vi "CPP_CalcTubingCorrection.vi"() -> (5 "Plug in titles":string[](array[string]), 7 "Plug in values":string[](array[string]))   [LabVIEW 2010]
uses:
  Globals/Plug_in_data_global.vi
  Globals/Meas_global.vi
  <vilib>/Analysis/NI_AALPro.lvlib
  <vilib>/Analysis/NI_AALBase.lvlib
panel:
  out "df":dbl format="%0.2f"
  out "Spectra":cluster{dbl, "df":dbl, dbl[][]}(graph)
  out "Current Block No":i32
  in  "stop":bool
  out "Time Traces":cluster{dbl, dbl, dbl[][]}(graph)
  in  "TestXducer":u16(ring) items=["Gen (Ref)", "Gen (t5w1)", "Gen (t2w2)", "Gen (t1w5)"]
  in  "RefXducer":u16(ring) items=["Gen (Ref)", "Gen (t5w1)", "Gen (t2w2)", "Gen (t1w5)"]
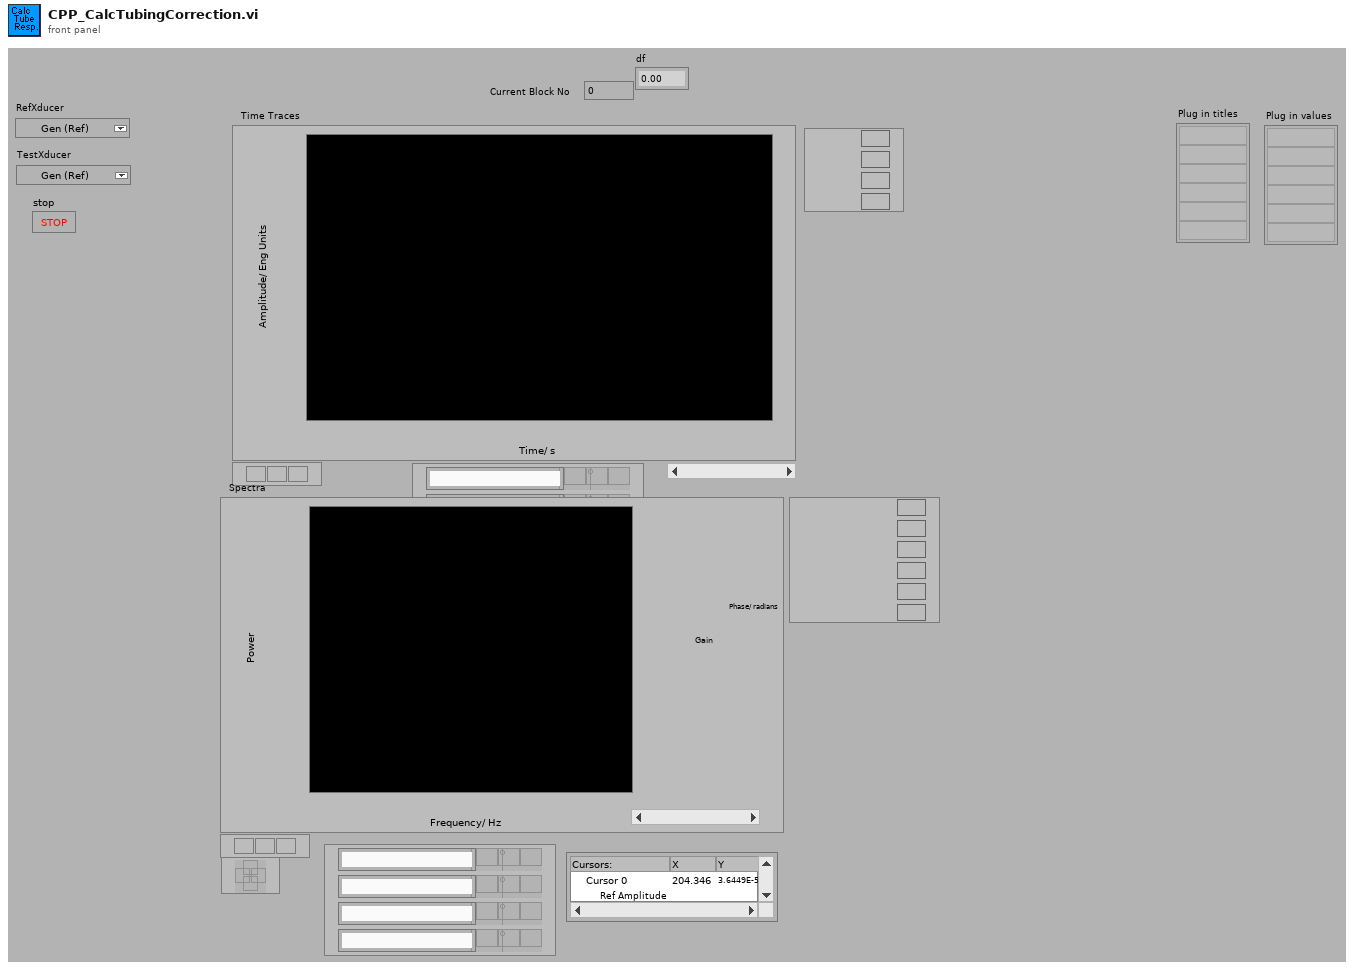
[diagram p1: front panel]
types:
  T1 = typedef "Analysis_info_cluster.ctl" = cluster{"Colour":u32, "Inst type":T2, "Inst name":string, "Symbol":string, "Code name":string, "Extra Info":string, "Inst Array":T3, "Index":i32, "Voltage Index":i32, "Extra Titles":string[], "Extra Values":string[]}
  T2 = typedef "Inst_type.ctl" = enum16{"Propeller anemometer", "Raw voltage", "Pressure Transducer", "Pitot-static tube", "Preston tube", "Hot wire", "Cross wire 1", "Cross wire 2", "Generic Linear", "Generic Polynomial", "Generic BackPoly", "Fast FID", "Thermocouple", "Cold wire", "Pulsed Wire", "LDA Vel", "LDA Tran time", "LDA Arr time"}
  T3 = typedef "Instrument_Array.ctl" = enum16{"PWA", "LDA", "Analogue"}
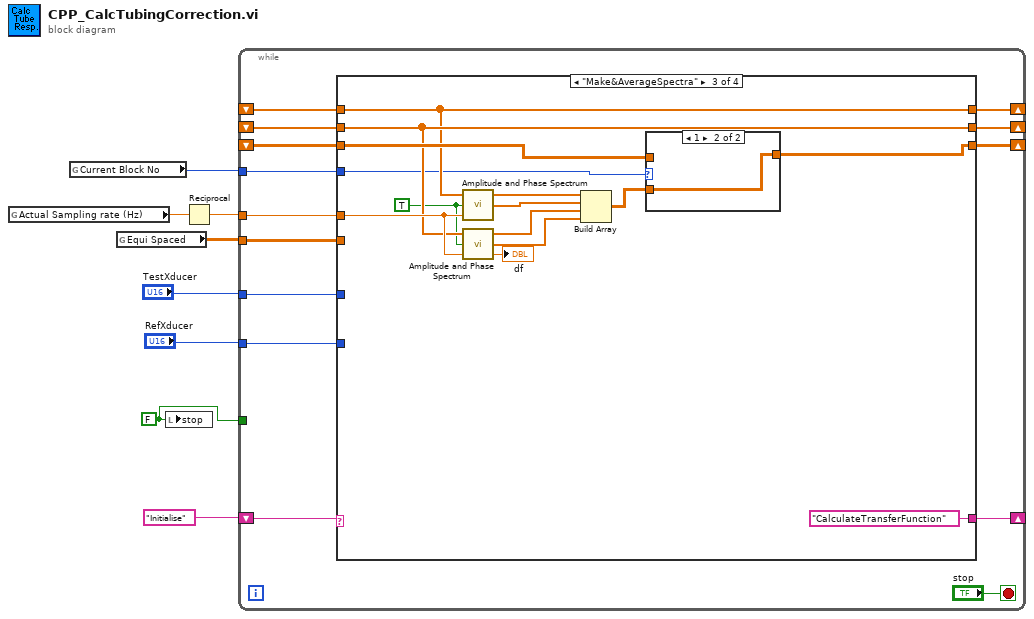
[diagram p0: block diagram]
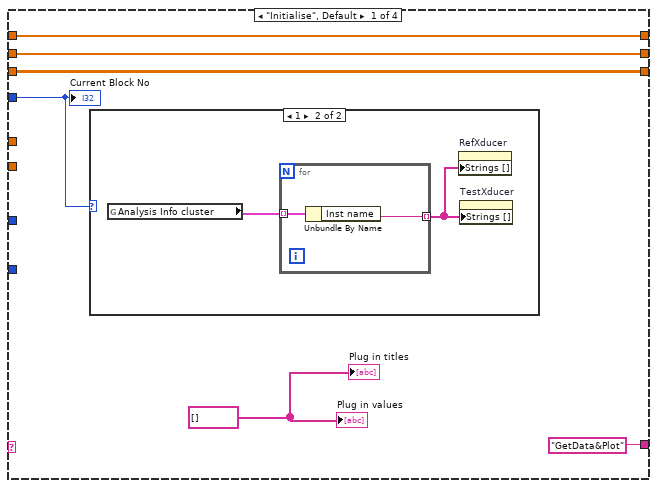
[diagram p2: hidden frame]
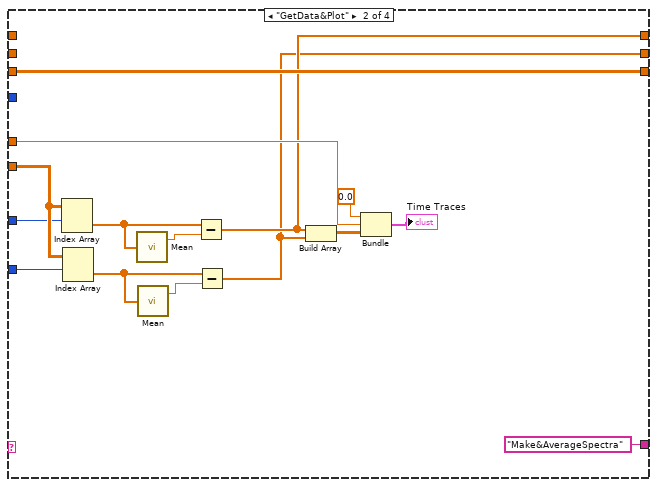
[diagram p4: hidden frame]
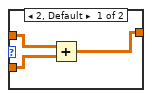
[diagram p5: hidden frame]
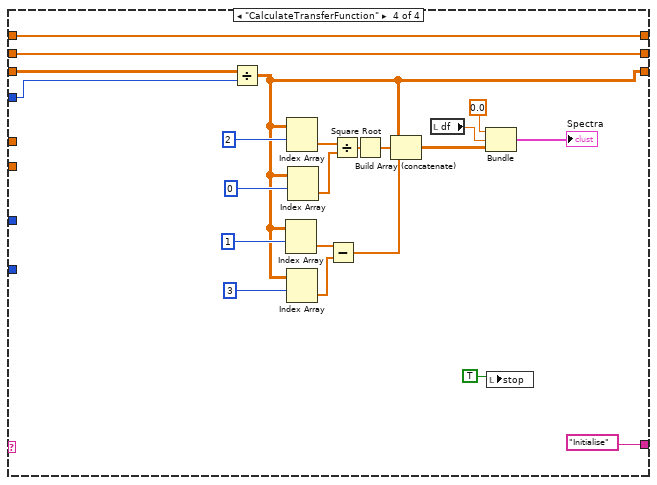
[diagram p6: hidden frame]
diagram:
  w6 = FALSE ("stop")
  n1 = global read "Meas_global.vi" "Actual Sampling rate (Hz)"() -> (w2:dbl)
  n2 = global read "Meas_global.vi" "Current Block No"() -> (w1:i32)
  n3 = global read "Plug_in_data_global.vi" "Equi Spaced"() -> (w7:dbl[][])
  n4 = local write "stop"(w6) -> ()
  n5 = Reciprocal(x=w2) -> (1/x=w3:dbl)
  n6 = while {
    shift-right: [w18] -> _
    shift-left: "Initialise" -> [w22]
    tunnel: w7 -> [w21]
    tunnel: "TestXducer" -> [w20]
    tunnel: "RefXducer" -> [w19]
    tunnel: w3 -> [w16]
    tunnel: w6 -> [_]
    shift-right: [w15] -> _
    shift-left: _ -> [w13]
    shift-right: [w14] -> _
    shift-left: _ -> [w12]
    shift-right: [w10] -> _
    shift-left: _ -> [w11]
    tunnel: w1 -> [w9]
    stop <- "stop" stop-if-true
    n7 = case shown="\"Make&AverageSpectra\"" w22 {
      tunnel: w21 -> [_ w47 _ _]
      tunnel: w20 -> [_ w46 _ _]
      tunnel: w19 -> [_ w45 _ _]
      tunnel: ["GetData&Plot" "Make&AverageSpectra" "CalculateTransferFunction" "Initialise"] -> w18
      tunnel: w16 -> [_ w40 w61 _]
      tunnel: [w26 w38 w55 w71] -> w15
      tunnel: [w25 w33 w56 w72] -> w14
      tunnel: w13 -> [w26 _ w55 w71]
      tunnel: w12 -> [w25 _ w56 w72]
      tunnel: w11 -> [w24 w39 w58 w80]
      tunnel: [w24 w39 w50 w73] -> w10
      tunnel: w9 -> [w23 _ w54 w79]
      frame "Initialise", Default {
        w28 = string[] [] ("Add in values")
        n8 = case shown="1" w23 {
          frame 0, Default {
          }
          frame 1 {
            n9 = global read "Meas_global.vi" "Analysis Info cluster"() -> (w29:T1[])
            n10 = for {
              tunnel: w29 -> [w32] mode=indexing
              tunnel: [w31] -> w30 mode=indexing
              n11 = Unbundle By Name(w32) -> ("Inst name"=w31:string)
            }
            n12 = property on="RefXducer" class="Ring (strict)"("Strings []"=w30) -> ()  [unwired: 2 in, 2 out]
            n13 = property on="TestXducer" class="Ring (strict)"("Strings []"=w30) -> ()  [unwired: 2 in, 2 out]
          }
        }
        "Plug in titles" <- w28
        "Plug in values" <- w28
        "Current Block No" <- w23
      }
      frame "GetData&Plot" {
        n14 = Index Array(array=w47, index (row)=w46) -> (element=w37:dbl[])  [unwired: 1 in]
        n15 = Index Array(array=w47, index (row)=w45) -> (element=w35:dbl[])  [unwired: 1 in]
        n16 = call <vilib>:"Mean.vi"("X"=w37) -> ("mean"=w36:dbl)  [unwired: 1 out]
        n17 = call <vilib>:"Mean.vi"("X"=w35) -> ("mean"=w34:dbl)  [unwired: 1 out]
        n18 = Subtract(x=w37, y=w36) -> (x-y=w38:dbl[])
        n19 = Subtract(x=w35, y=w34) -> (x-y=w33:dbl[])
        n20 = Build Array(w38, w33) -> (w43:dbl[][])
        n21 = Bundle(0.0, w40, w43) -> (→"Time Traces":cluster{dbl, dbl, dbl[][]})  [unwired: 1 in]
      }
      frame "Make&AverageSpectra" {
        w53 = TRUE ("unwrap phase (T)")
        n22 = call <vilib>:"Amplitude and Phase Spectrum.vi"("dt"=w61, "unwrap phase (T)"=w53, "Signal (V)"=w55) -> ("Amp Spectrum Phase (radians)"=w51:dbl[], "Amp Spectrum Mag (Vrms)"=w60:dbl[])  [unwired: 1 out]
        n23 = call <vilib>:"Amplitude and Phase Spectrum.vi"("dt"=w61, "unwrap phase (T)"=w53, "Signal (V)"=w56) -> ("df"=→"df":dbl, "Amp Spectrum Phase (radians)"=w52:dbl[], "Amp Spectrum Mag (Vrms)"=w59:dbl[])
        n24 = Build Array(w60, w51, w59, w52) -> (w57:dbl[][])
        n25 = case shown="1" w54 {
          tunnel: w58 -> [w64 _]
          tunnel: w57 -> [w63 w65]
          tunnel: [w62 w65] -> w50
          frame 2, Default {
            n26 = Add(x=w64, y=w63) -> (x+y=w62:dbl[][])
          }
          frame 1 {
          }
        }
      }
      frame "CalculateTransferFunction" {
        n27 = Divide(x=w80, y=w79) -> (x/y=w73:dbl[][])
        n28 = Index Array(array=w73, index (row)=1) -> (element=w85:dbl[])  [unwired: 1 in]
        n29 = Index Array(array=w73, index (row)=2) -> (element=w75:dbl[])  [unwired: 1 in]
        n30 = Index Array(array=w73, index (row)=3) -> (element=w84:dbl[])  [unwired: 1 in]
        n31 = Index Array(array=w73, index (row)=0) -> (element=w74:dbl[])  [unwired: 1 in]
        n32 = Subtract(x=w85, y=w84) -> (x-y=w69:dbl[])
        n33 = Divide(x=w75, y=w74) -> (x/y=w70:dbl[])
        n34 = Square Root(x=w70) -> (sqrt(x)=w66:dbl[])
        n35 = Build Array (concatenate)(w73, w66, w69) -> (w81:dbl[][])
        n36 = local read "df"() -> (w78:dbl)
        n37 = Bundle(0.0, "df"=w78, w81) -> (→"Spectra":cluster{dbl, "df":dbl, dbl[][]})  [unwired: 1 in]
        n38 = local write "stop"(TRUE ("stop")) -> ()
      }
    }
  }
